vi "LV Graph to Igor UI.vi"() -> ()   [LabVIEW 2019, in "LV-Data.ITX.lvclass"]
uses:
  LV-Data.ITX.lvclass
panel:
  in  "write file?":bool
  in  "X,Y,Z Scale Names":string[](array[string])=["X", "Y", "Z"]
  in  "Enum":enum16{"XY Graph", "Intensity Graph"}(ring)
  out "Tab":enum32{"XY Graph", "Intensity Graph"}(tab)
  in  "XY Graph":cluster{dbl[], dbl[]}[](graph)
  in  "Intensity Graph":dbl[][](graph)
  in  "Path":path=path "C:/temp"
  in  "Filename":string="testname"
  in  "open file in Igor?":bool
  # "<-- choose which graph you would like to save"
  # "Igor Syntax:\n\\S = superscript\n\\B = subscript\n\\M = normal\n\nExample:\nV\\MS\\B = \"V_S\""
  # "adjust offset and multiplier\nhere to make your graph look\ncorrect in Igor"
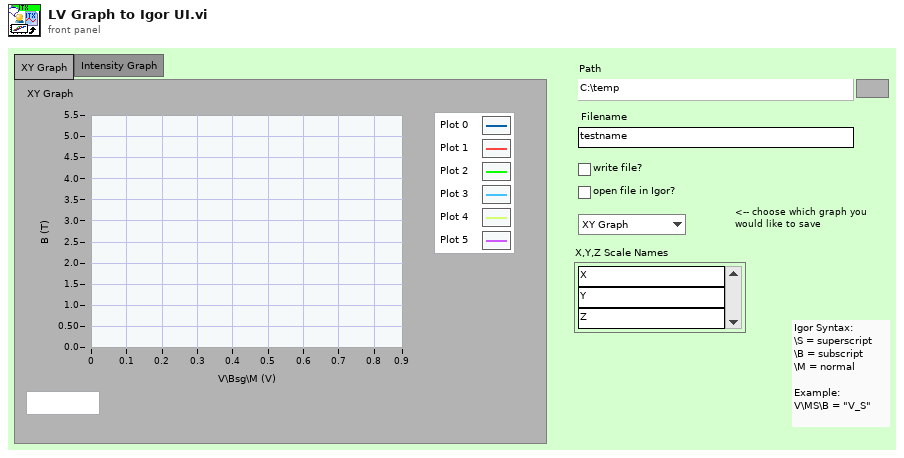
[diagram p1: front panel]
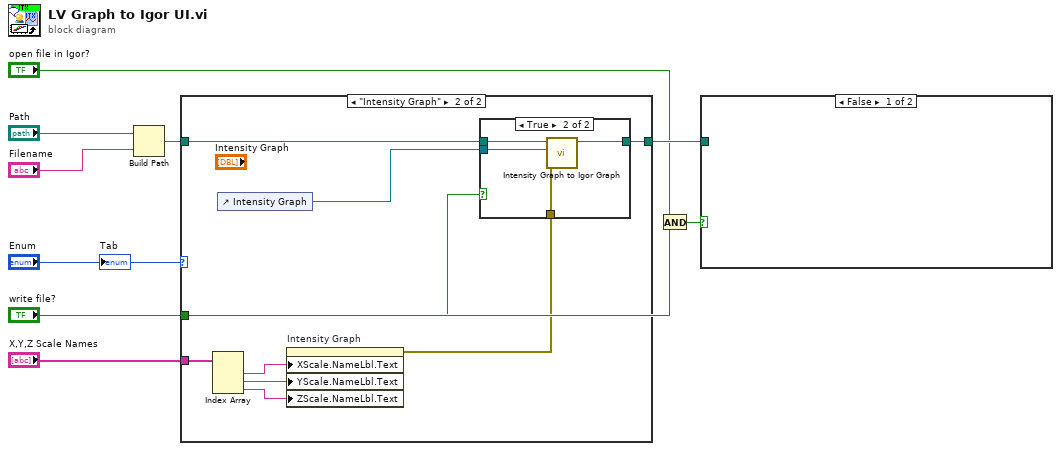
[diagram p0: block diagram]
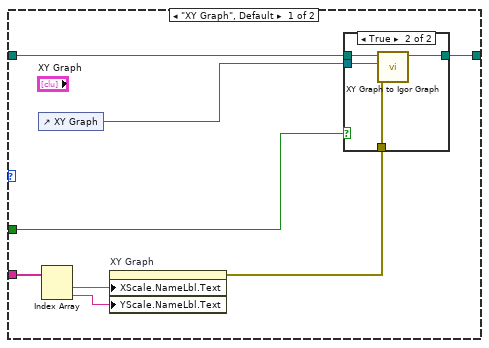
[diagram p2: hidden frame]
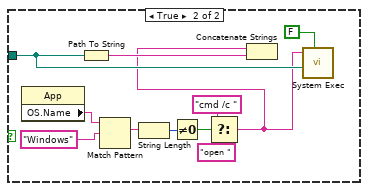
[diagram p5: hidden frame]
diagram:
  n1 = Build Path(base path="Path", name or relative path="Filename") -> (appended path=w6:path)
  n2 = case shown="\"Intensity Graph\"" "Enum" {
    tunnel: w6 -> [w17 w30]
    tunnel: [w16 w31] -> w9
    tunnel: "X,Y,Z Scale Names" -> [w15 w29]
    tunnel: "write file?" -> [w10 w23]
    frame "XY Graph", Default {
      n3 = control-ref of="XY Graph"() -> (w12:refnum<vi>)
      n4 = Index Array(array=w15) -> (element #1=w14:string, element #2=w13:string)  [unwired: 2 in]
      n5 = property on="XY Graph" class="XYGraph (strict)"("XScale.NameLbl.Text"=w14, "YScale.NameLbl.Text"=w13) -> (error out=w11:errorcluster)  [unwired: 2 in, 1 out]
      n6 = case shown="True" w10 {
        tunnel: w17 -> [w18 w21]
        tunnel: [w18 w20] -> w16
        tunnel: w12 -> [_ w22]
        tunnel: w11 -> [_ w19]
        frame False {
        }
        frame True {
          n7 = call "XY Graph to Igor Graph.vi"("error in (no error)"=w19, "XY Graph Reference"=w22, "Path"=w21) -> ("file"=w20:path)  [unwired: 7 in, 1 out]
        }
      }
    }
    frame "Intensity Graph" {
      n8 = Index Array(array=w29) -> (element #1=w27:string, element #2=w28:string, element #3=w26:string)  [unwired: 3 in]
      n9 = control-ref of="Intensity Graph"() -> (w24:refnum<vi>)
      n10 = property on="Intensity Graph" class="IntGraph (strict)"("XScale.NameLbl.Text"=w27, "YScale.NameLbl.Text"=w28, "ZScale.NameLbl.Text"=w26) -> (error out=w25:errorcluster)  [unwired: 2 in, 1 out]
      n11 = case shown="True" w23 {
        tunnel: [w32 w35] -> w31
        tunnel: w30 -> [w32 w36]
        tunnel: w25 -> [_ w34]
        tunnel: w24 -> [_ w33]
        frame False {
        }
        frame True {
          n12 = call "Intensity Graph to Igor Graph.vi"("error in (no error)"=w34, "Intensity Graph Reference"=w33, "Path"=w36) -> ("file"=w35:path)  [unwired: 7 in, 1 out]
        }
      }
    }
  }
  n13 = And(x="open file in Igor?", y="write file?") -> (x .and. y?=w1:bool)
  n14 = case shown="False" w1 {
    tunnel: w9 -> [_ w38]
    frame False {
    }
    frame True {
      n15 = property class="App"() -> ("OS.Name"=w41:string)  [unwired: 2 in, 2 out]
      n16 = Path To String(path=w38) -> (string=w39:string)
      n17 = Match Pattern(string=w41, regular expression="Windows") -> (match substring=w47:string)  [unwired: 1 in, 3 out]
      n18 = String Length(string=w47) -> (length=w46:i32)
      n19 = Not Equal To 0?(x=w46) -> (x != 0?=w44:bool)
      n20 = Select(t="cmd /c ", s=w44, f="open ") -> (s? t:f=w37:string)
      n21 = Concatenate Strings(w37, w39) -> ()  [unwired: 1 out]
      n22 = call <vilib>:"System Exec.vi"("wait until completion? (T)"=FALSE, "working directory"=w38, "command line"=w37) -> ()  [unwired: 5 in, 4 out]
    }
  }
  "Tab" <- "Enum"
